vi "setChannel.vi"(8 "error in (no error)":errorcluster, 10 "Channel.lvclass":refnum<class "Channel.lvclass">, 11 "rf.lvclass in":refnum<class "rf.lvclass">) -> (0 "error out":errorcluster, 3 "rf.lvclass out":refnum<class "rf.lvclass">)   [LabVIEW 2009, in "Tools.lvlib" / "Scripting.lvlib" / "rf.lvclass"]
uses:
  rf.lvclass
  DatabaseHelpers/Database Objects/Channel/Channel.lvclass
  ScriptEvent.lvclass
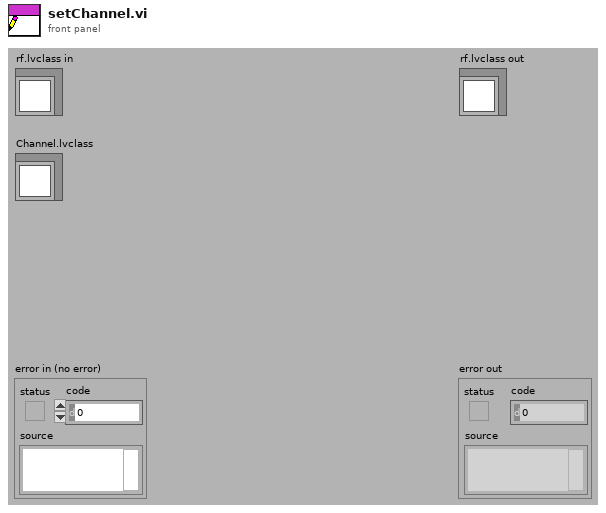
[diagram p1: front panel]
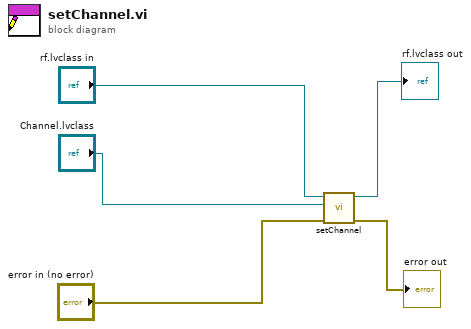
[diagram p0: block diagram]
diagram:
  n1 = call-parent "setChannel.vi"("error in (no error)"="error in (no error)", "Channel.lvclass"="Channel.lvclass", "ScriptEvent.lvclass in"="rf.lvclass in") -> ("error out"=→"error out":errorcluster, "ScriptEvent.lvclass out"=→"rf.lvclass out":refnum<class "rf.lvclass">)  [unwired: 7 in]
